vi "Error_Handler.vi"(7 "error mode":T2(ring)=enum."Check Error", 8 "error in":errorcluster, 10 "Error event ref":refnum<user-event>, 11 "Queue Ref in":T1[](array[typedef])) -> (0 "error out":errorcluster, 2 "Error event ref out":refnum<user-event>, 3 "Queue Ref out":T1[](array[typedef]))   [LabVIEW 2019]
doc: "Error Handler Module Template\n\nThis vi is used to handle error info, especially for parallel loops. It consists three mode:\n\n1. Initialize mode is to initiallize error cluster array and any queue ref, user event ref, or timedloop name that will be used to stop parallel loops\n2. Check Error mode is the main operation for this vi. If the status of error in is true, determine whether the size of error array is ZERO, namely no error happens before, then add new error to the error array. If this is the first error, clear error and stop parallel loops using enqueue function or generate user event function with error cluster type; otherwise just add new error to error array.\n3. Report Error mode is to output error cluster with Merge Errors function.\n\nChenny Wang"
uses:
  core/core_dataRef.ctl
  core/core_dataCluster.ctl
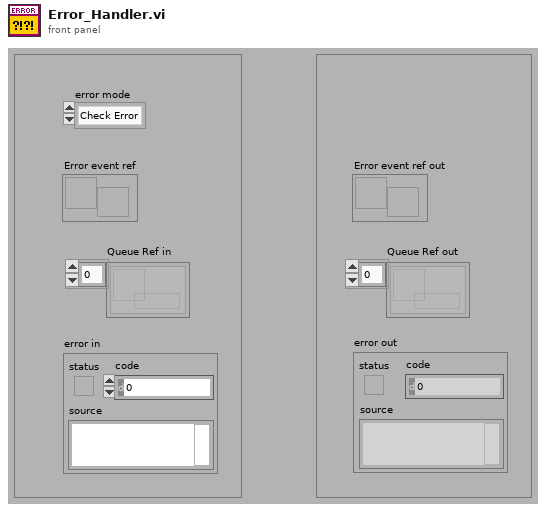
[diagram p1: front panel]
types:
  T1 = typedef "core_dataRef.ctl" = refnum<queue>
  T2 = enum16{"Initialize", "Check Error", "Report Error"}
  T3 = typedef "core_dataCluster.ctl" = cluster{"cmd":string, "data":variant}
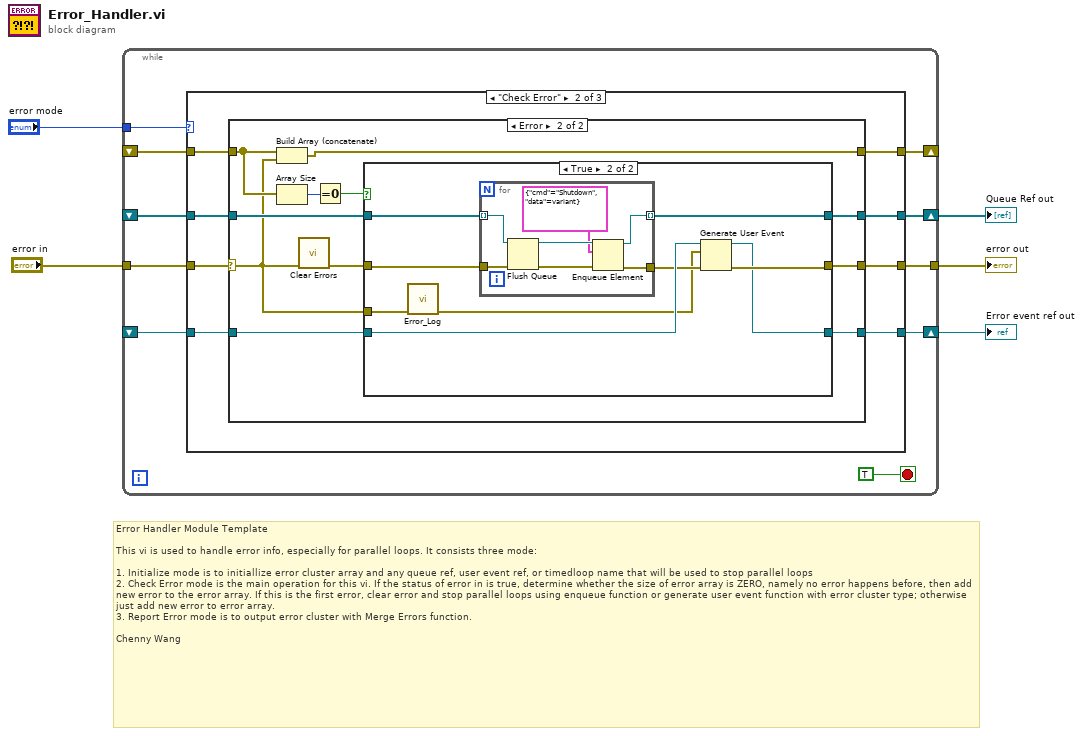
[diagram p0: block diagram]
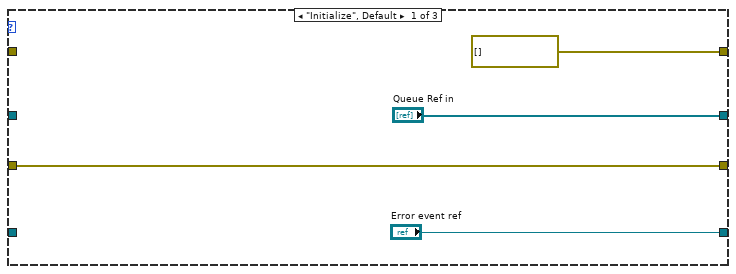
[diagram p2: hidden frame]
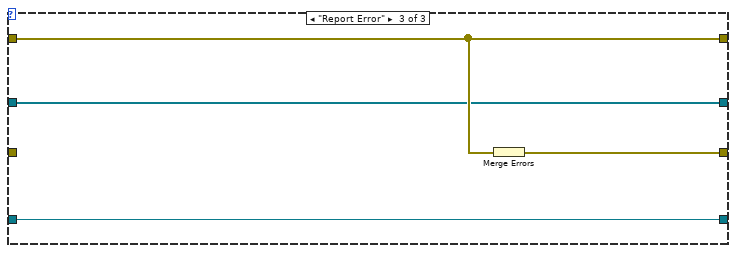
[diagram p5: hidden frame]
diagram:
  # "Error Handler Module Template\n\nThis vi is used to handle error info, especially for parallel loops. It consists three mode:\n\n1. Initialize mode is to initiallize error cluster array and any queue ref, user event ref, or timedloop name that will be used to stop parallel loops\n2. Check Error mode is the main operation for this vi. If the status of error in is true, determine whether the size of error array is ZERO, namely no error happens before, then add new error to the error array. If this is the first error, clear error and stop parallel loops using enqueue function or generate user event function with error cluster type; otherwise just add new error to error array.\n3. Report Error mode is to output error cluster with Merge Errors function.\n\nChenny Wang"
  n1 = while {
    tunnel: "error mode" -> [w14]
    shift-right: [w13] -> _
    shift-left: _ -> [w12]
    tunnel: "error in" -> [w11]
    tunnel: [w10] -> w3
    shift-right: [w9] -> w1
    shift-left: _ -> [w7]
    shift-right: [w8] -> w2
    shift-left: _ -> [w6]
    stop <- TRUE stop-if-true
    n2 = case shown="\"Check Error\"" w14 {
      tunnel: [errorcluster[] [] w25 w65] -> w13
      tunnel: w12 -> [_ w26 w65]
      tunnel: w11 -> [w18 w27 _]
      tunnel: [w18 w24 w64] -> w10
      tunnel: ["Queue Ref in" w20 w63] -> w9
      tunnel: ["Error event ref" w21 w62] -> w8
      tunnel: w7 -> [_ w23 w63]
      tunnel: w6 -> [_ w22 w62]
      frame "Initialize", Default {
      }
      frame "Check Error" {
        n3 = case shown="Error" w27 {
          selector: w27 -> [w30 w32]
          tunnel: w26 -> [w31 w40]
          tunnel: [w31 w39] -> w25
          tunnel: [w30 w37] -> w24
          tunnel: w23 -> [w29 w36]
          tunnel: w22 -> [w28 w35]
          tunnel: [w28 w34] -> w21
          tunnel: [w29 w33] -> w20
          frame No Error {
          }
          frame Error {
            n4 = Build Array (concatenate)(w40, w32) -> (w39:errorcluster[])
            n5 = Array Size(array=w40) -> (size(s)=w42:i32)
            n6 = call <vilib>:"Clear Errors.vi"("error in (no error)"=w32) -> ("error out"=w38:errorcluster)  [unwired: 5 in, 1 out]
            n7 = Equal To 0?(x=w42) -> (x = 0?=w41:bool)
            n8 = case shown="True" w41 {
              tunnel: w38 -> [w45 w54]
              tunnel: [w45 w52] -> w37
              tunnel: w36 -> [w44 w53]
              tunnel: w35 -> [w43 w50]
              tunnel: [w43 w49] -> w34
              tunnel: [w44 w51] -> w33
              tunnel: w32 -> [_ w47]
              frame False {
              }
              frame True {
                n9 = call "Error_Log.vi"("error in (no error)"=w47) -> ("error out"=w46:errorcluster)  [unwired: 10 in]
                n10 = for {
                  tunnel: w54 -> [w61]
                  tunnel: w53 -> [w60] mode=indexing
                  tunnel: [w57] -> w48
                  tunnel: [w56] -> w51 mode=indexing
                  n11 = Flush Queue(queue=w60, error in (no error)=w61) -> (queue out=w58:T1, error out=w59:errorcluster)  [unwired: 1 out]
                  n12 = Enqueue Element(queue=w58, element=T3 {"cmd"="Shutdown", "data"=variant}, error in (no error)=w59) -> (queue out=w56:T1, error out=w57:errorcluster)  [unwired: 1 in, 1 out]
                }
                n13 = Generate User Event(user event=w50, event data cluster=w46, error in=w48) -> (user event out=w49:refnum<user-event>, error out=w52:errorcluster)  [unwired: 1 in]
              }
            }
          }
        }
      }
      frame "Report Error" {
        n14 = Merge Errors(w65) -> (w64:errorcluster)
      }
    }
  }
  "error out" <- w3
  "Error event ref out" <- w2
  "Queue Ref out" <- w1
